vi "scheduler.vi"(11 "Name (\"\" to Use UUID)":string) -> ()   [LabVIEW 2025]
uses:
  supports/Waypoint.ctl
  d7dd9159-89a2-4514-95bd-649e26e943bd.vi
  <vilib>/numeric/Random Number (Range) I64.vi
  49f21eb9-f673-4fa8-8715-351f05abaff7.vi
  0d6ab66a-5149-4c79-b89e-f55ee53f3b39.vi
  3f08c095-eb42-4770-a6b1-2c55b3203edd.vi
  cd06cb13-84a1-4604-9614-019e20008b86.vi
  <userlib>/_NEVSTOP/Communicable State Machine(CSM)/AdvanceAPI/CSM - Revert Arguments-Safe String.vi
  <userlib>/_NEVSTOP/Communicable State Machine(CSM)/AdvanceAPI/CSM - Make String Arguments Safe.vi
  <userlib>/_NEVSTOP/Communicable State Machine(CSM)/AdvanceAPI/CSM - Break Down Multiple States String.vi
  <userlib>/_NEVSTOP/Communicable State Machine(CSM)/AdvanceAPI/CSM - Compact Multiple States.vi
  <vilib>/numeric/sub_Random U32.vi
  <userlib>/_NEVSTOP/Communicable State Machine(CSM)/AdvanceAPI/CSM - Keywords.vi
  <userlib>/_NEVSTOP/Communicable State Machine(CSM)/_Shared/Trim Single-line Text.vi
  <userlib>/_NEVSTOP/Communicable State Machine(CSM)/addons/MassData-Parameter/_support/FGV-MassData(lvlibp).vi
  <userlib>/_NEVSTOP/Communicable State Machine(CSM)/_Polymophic/Build Status Broadcast Message.vi
  <userlib>/_NEVSTOP/Communicable State Machine(CSM)/Communicable State Machine.lvlib
panel:
  out "Trajectory":cluster{"x":i32, "y":i32}[](graph)
  out "Path":T1[](graph)=[{"x"=0, "y"=0}, {"x"=-1, "y"=0}]
  out "Error Occurred":errorcluster
  out "State History":string
  in  "Exit":bool
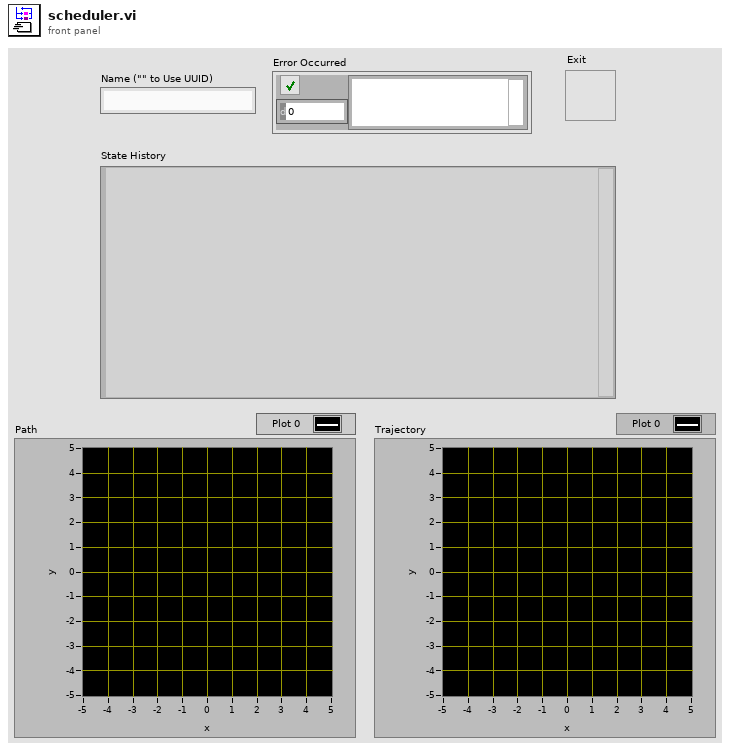
[diagram p1: front panel]
types:
  T1 = typedef "Waypoint.ctl" = cluster{"x":i32, "y":i32}
  T2 = enum32{"Invalid", "Standard", "Closed", "Hidden", "Minimized", "Maximized"}
  T3 = enum32{"invalid app kind", "Development System", "Run Time System", "Student Edition", "Embedded LabVIEW", "Evaluation", "Custom"}
  T4 = typedef "Communicable State Machine.lvlib/_CSM_Response Source Message.ctl" = cluster{"‘State":string, "’Arguments":string, "’Error":errorcluster}
  T5 = cluster{"Current VI Reference":refnum<vi>, "Close Panel on Exit?":bool}
  T6 = cluster{"Core":cluster{"Current VI Reference":refnum<vi>, "Close Panel on Exit?":bool}, "Level":i32, "Path":T1[], "Waypoint":T1}
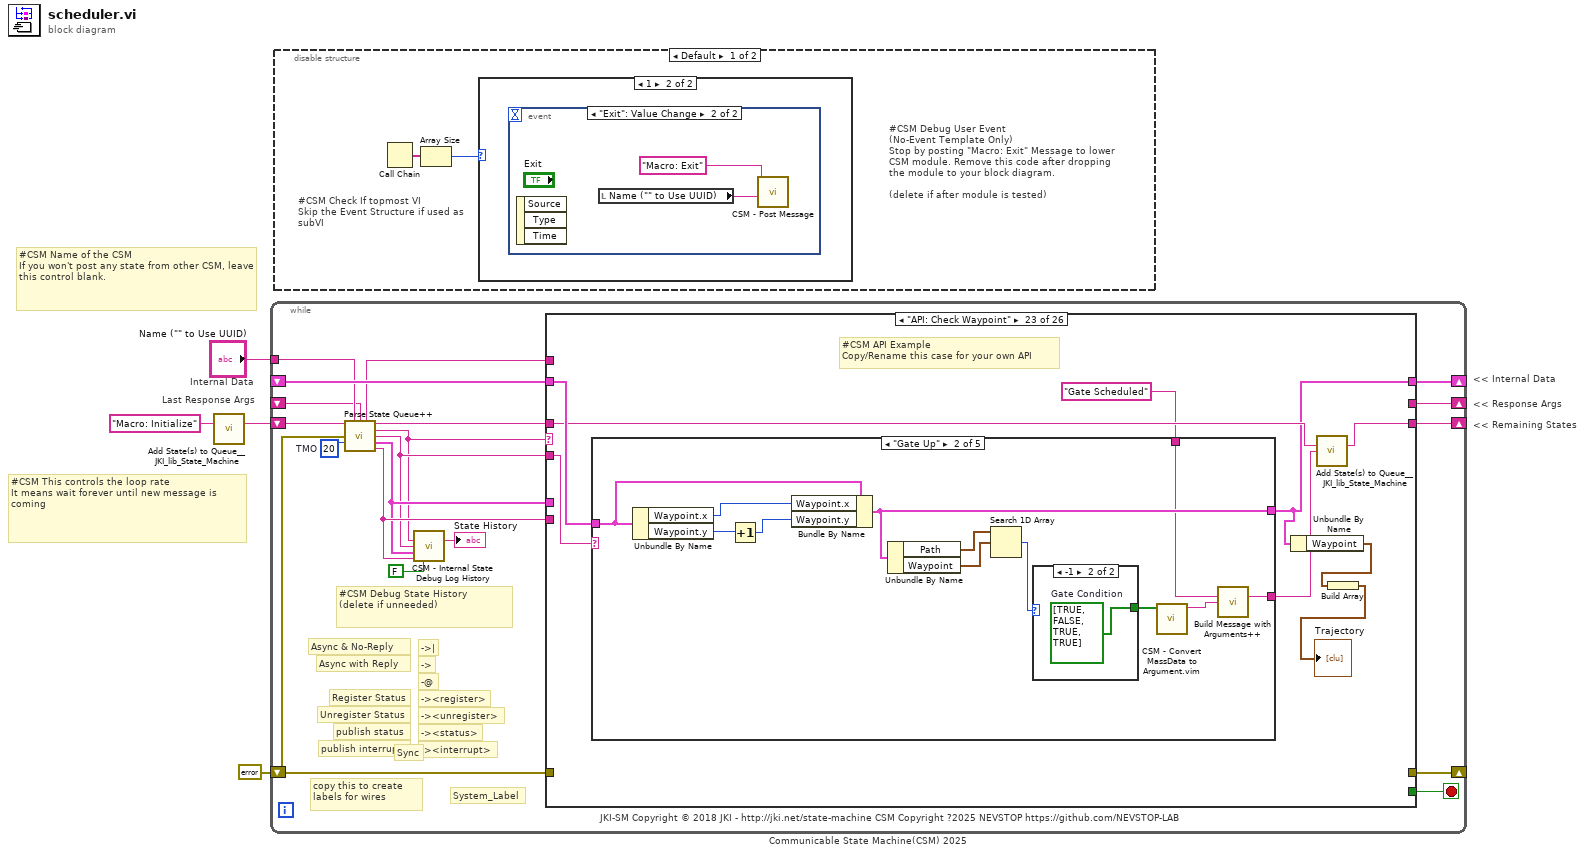
[diagram p0: block diagram]
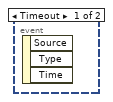
[diagram p3: hidden frame]
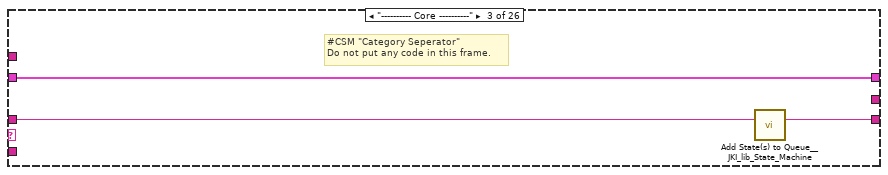
[diagram p7: hidden frame]
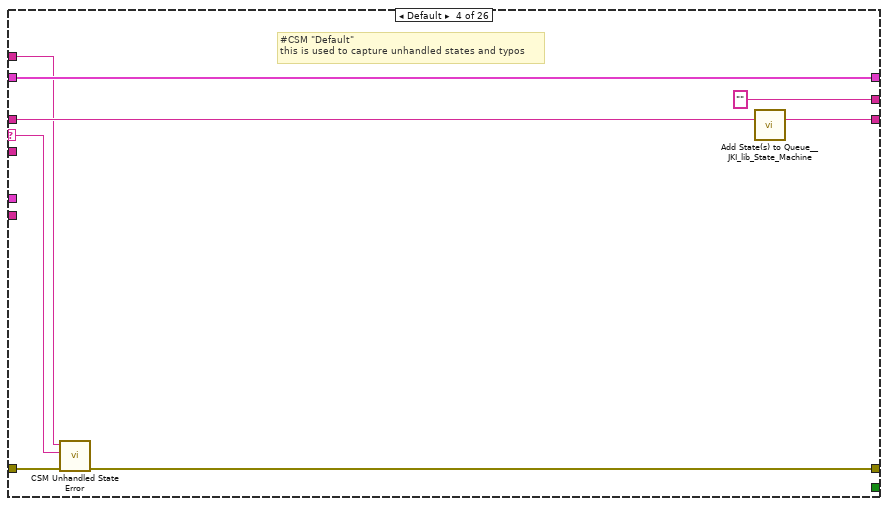
[diagram p8: hidden frame]
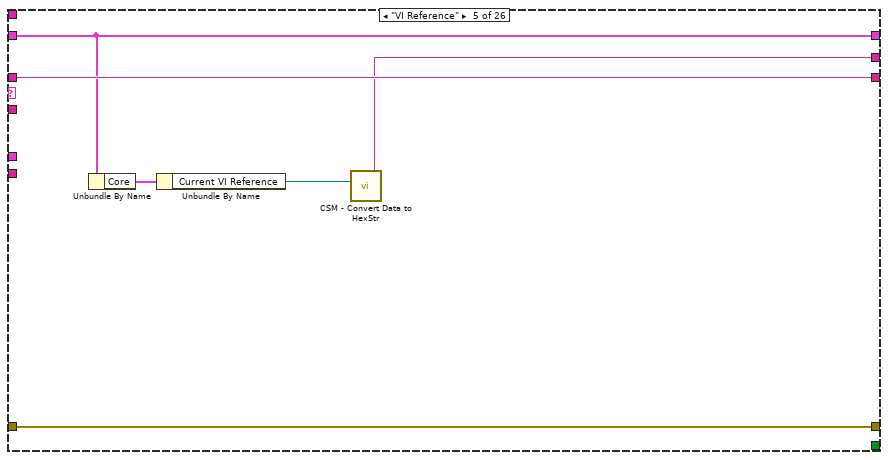
[diagram p9: hidden frame]
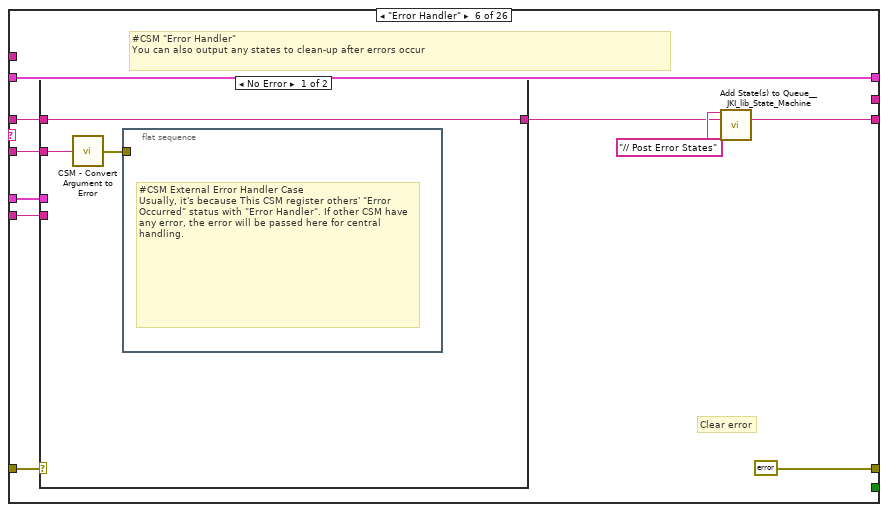
[diagram p10: hidden frame]
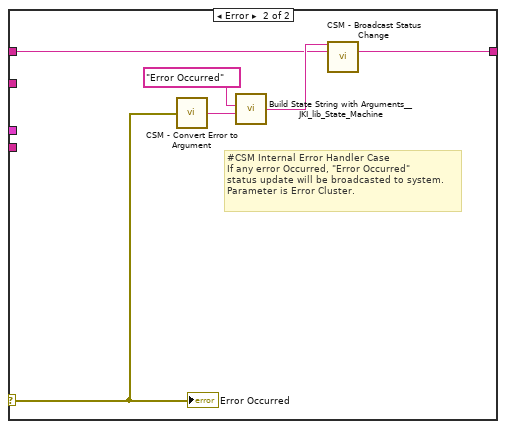
[diagram p11: hidden frame]
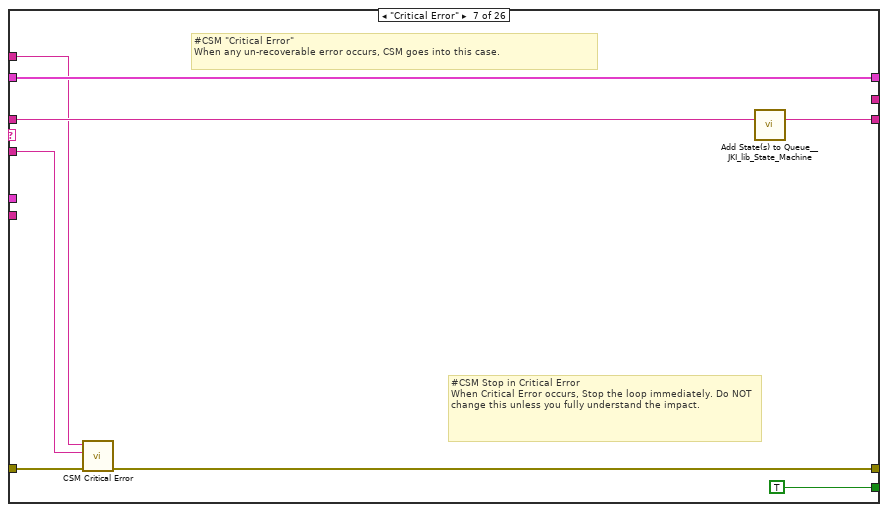
[diagram p12: hidden frame]
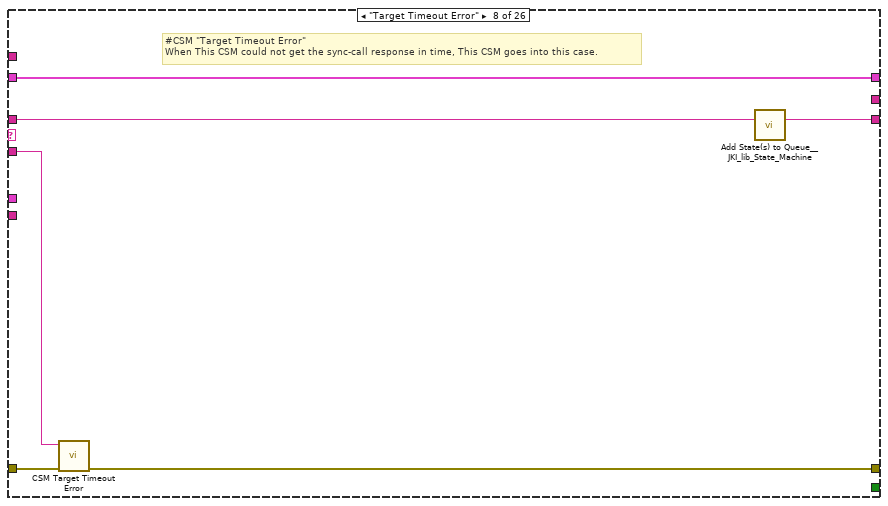
[diagram p13: hidden frame]
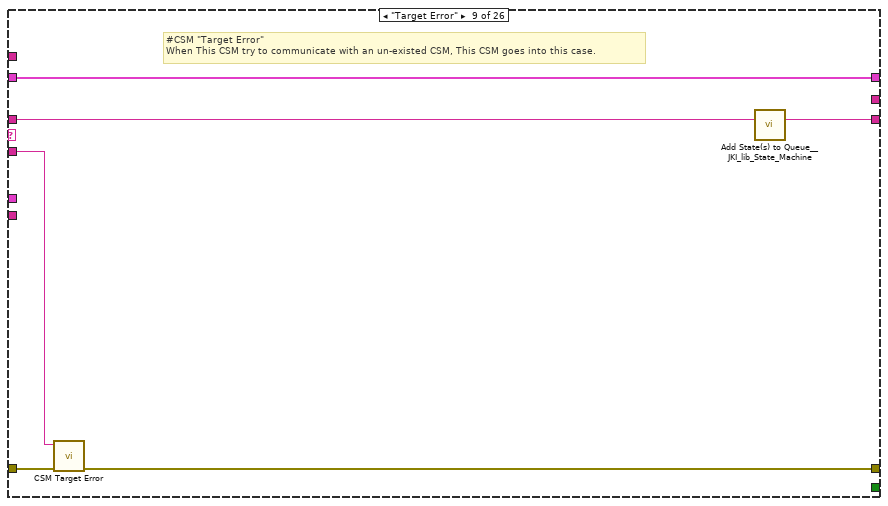
[diagram p14: hidden frame]
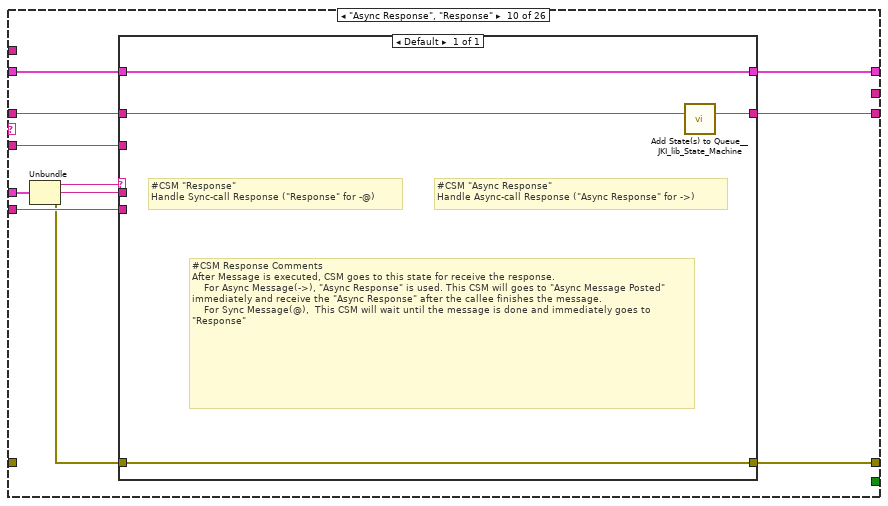
[diagram p15: hidden frame]
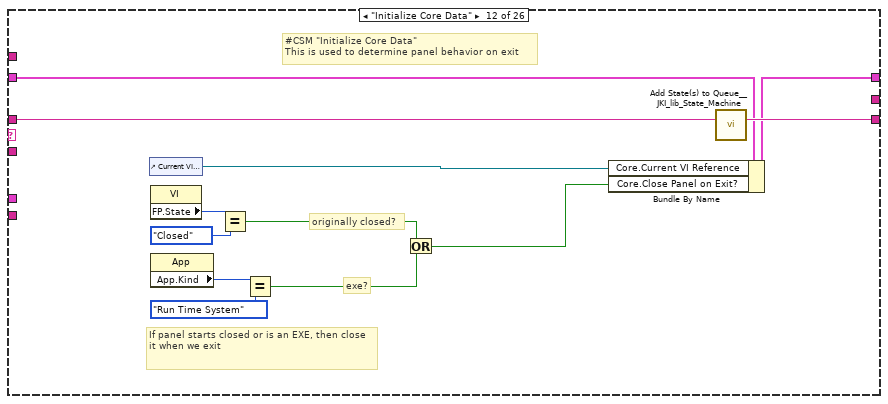
[diagram p17: hidden frame]
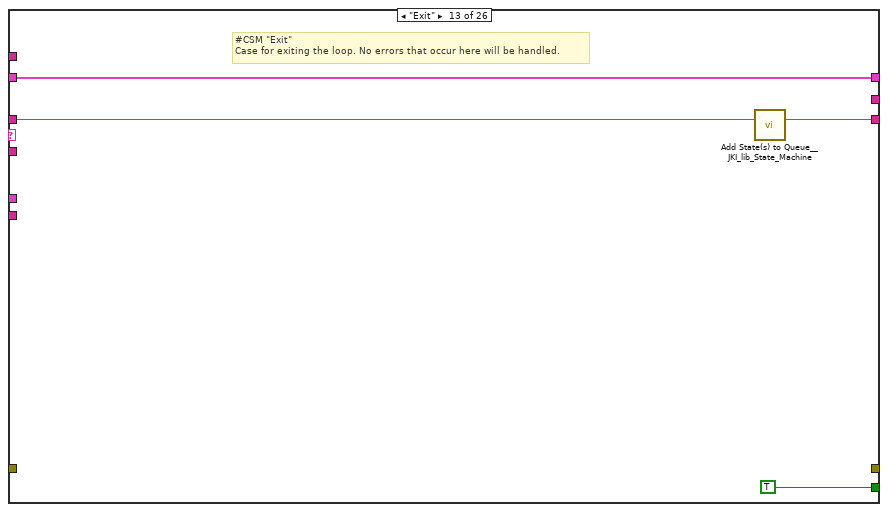
[diagram p18: hidden frame]
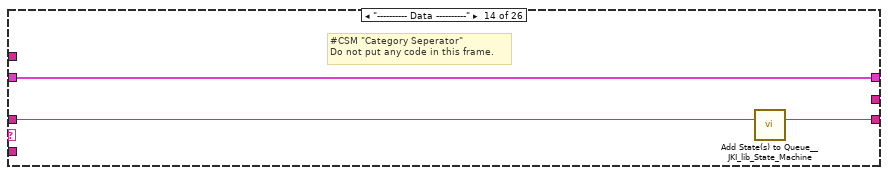
[diagram p19: hidden frame]
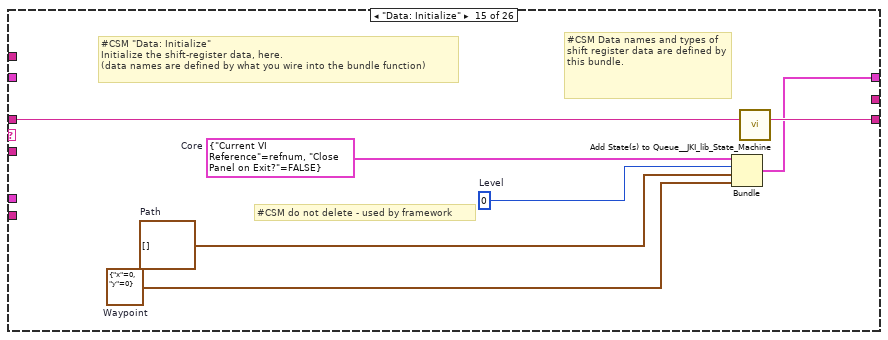
[diagram p20: hidden frame]
diagram:
  # "Last Response Args"
  # "Internal Data"
  # "#CSM Name of the CSM\nIf you won't post any state from other CSM, leave this control blank."
  # "#CSM This controls the loop rate\nIt means wait forever until new message is coming"
  # "<< Internal Data"
  # "<< Response Args"
  # "<< Remaining States"
  n1 = call <vilib>:"Add State(s) to Queue__JKI_lib_State_Machine.vi"("State(s) in (\"\")"="Macro: Initialize" ("Init State(\"Macro: Initialize\")")) -> ("States Out"=w1:string)  [unwired: 14 in]
  n2 = while "Communicable State Machine(CSM) 2025" {
    shift-right: [w18] -> _
    shift-left: _ -> [w17]
    shift-right: [w21] -> _
    shift-left: errorcluster {"status"=FALSE, "code"=0, "source"=""} ("error out") -> [w7]
    shift-right: [w20] -> _
    shift-left: w1 -> [w22]
    tunnel: "Name (\"\" to Use UUID)" -> [w14]
    shift-right: [w15] -> _
    shift-left: _ -> [w9]
    stop <- w19 stop-if-true
    w16 = 20  # TMO
    # "#CSM Debug State History\n(delete if unneeded)"
    # "-><interrupt>"
    # "-><status>"
    # "-><unregister>"
    # "-><register>"
    # "-@"
    # "->"
    # "->|"
    # "publish interrupt"
    # "publish status"
    # "Unregister Status"
    # "Register Status"
    # "Sync"
    # "Async with Reply"
    # "Async & No-Reply"
    # "JKI-SM Copyright © 2018 JKI - http://jki.net/state-machine CSM Copyright ?2025 NEVSTOP https://github.com/NEVSTOP-LAB"
    # "copy this to create labels for wires"
    # "System_Label"
    n3 = call <userlib>:"Parse State Queue++.vi"("State Queue"=w22, "Name (\"\" to Use UUID)"=w14, "Response Arguments"=w9, "Previous Error"=w7, "Dequeue (1 ms)"=w16) -> ("Name Used"=w8:string, "Remaining States"=w23:string, "Current State"=w10:string, "Arguments"=w11:string, "Additional Information"=w12:T4, "Source CSM"=w13:string)  [unwired: 5 in]
    n4 = call <userlib>:"CSM - Internal State Debug Log History.vi"("State"=w10, "Arguments (\"\")"=w11, ">> Response Source Message >>"=w12, "Source (\"\")"=w13, "Enable Periodic State Filter? (T)"=FALSE) -> ("Debug Log"=→"State History":string)  [unwired: 10 in]
    n5 = case shown="\"API: Check Waypoint\"" w10 {
      selector: w10 -> [_ _ _ w34 _ _ _ _ _ _ _ _ _ _ _ _ _ _ _ _ _ _ _ _ _ _]
      tunnel: w23 -> [w24 w27 w30 w38 w43 w48 w71 w77 w83 w93 w100 w112 w116 w119 w126 w128 w134 w137 w141 w147 w149 w159 w225 w288 w291 w294]
      tunnel: w11 -> [_ _ _ _ _ w47 w67 w74 w80 w87 _ _ _ _ _ _ _ _ _ _ _ w155 w227 _ _ _]
      tunnel: w17 -> [w25 w26 w28 w36 w42 w53 w69 w75 w81 w91 w99 w106 w114 w117 _ w127 w129 w135 w139 w145 w148 w158 w226 w286 w289 w292]
      tunnel: [_ _ _ w31 w44 errorcluster {"status"=FALSE, "code"=0, "source"=""} ("error out") w64 w72 w78 w94 _ _ _ _ _ _ w130 _ _ _ _ _ _ _ _ _] -> w21
      tunnel: w7 -> [_ _ _ w32 w44 w51 w65 w73 w79 _ _ _ _ _ _ _ w131 _ _ _ _ _ _ _ _ _]
      tunnel: [w24 w27 w29 w37 w43 w49 w70 w76 w82 w92 w100 w111 w115 w118 w125 w128 w133 w136 w140 w146 w149 w159 w224 w287 w290 w293] -> w20
      tunnel: [_ _ _ _ _ _ TRUE _ _ _ _ _ TRUE _ _ _ _ _ _ _ _ _ _ _ _ _] -> w19
      tunnel: [w25 w26 w28 w36 w42 w53 w69 w75 w81 w90 w99 w110 w114 w117 w124 w127 w129 w135 w139 w145 w148 w157 w221 w286 w289 w292] -> w18
      tunnel: w13 -> [_ _ _ _ _ w46 _ _ _ w88 _ _ _ _ _ _ _ _ _ _ _ _ _ _ _ _]
      tunnel: w12 -> [_ _ _ _ _ w45 _ _ _ w89 _ _ _ _ _ _ _ _ _ _ _ _ _ _ _ _]
      tunnel: [_ _ _ "" w39 _ _ _ _ _ _ _ _ _ _ _ _ _ _ _ _ "Scheduler Began" ("HEX String (0-9,A-F)") _ _ _ _] -> w15
      tunnel: w8 -> [_ _ _ w33 _ _ w66 _ _ _ _ _ _ _ _ _ _ _ _ _ _ _ _ _ _ _]
      frame "", "Idle" {
        # "#CSM \"Idle/Event Handler\"\nexecutes when the state queue is empty"
      }
      frame "CSM Documentation" {
        # "#CSM State Syntax\n\n// Comment line, all text to the right of “//” will be ignored\n// Local Message Example\nDoSth: DoA >> Arguments\n\n// Sync Call Example\nAPI: xxxx >> Arguments -@ TargetModule\n\n// Async Call Example\nAPI: xxxx >> Arguments -> TargetModule\n\n// Async Call without Reply Example\nAPI: xxxx >> Arguments ->| TargetModule\n\n// Broadcast normal status:\nStatus >> StatusArguments  -><status>\n\n// Broadcast Interrupt status:\nInterrupt >> StatusArguments  -><interrupt>\n\n// Register Source Module's status to Handler Module\nStatus@Source Module >> Handler Module@Handler Module -><register>\n\n// Unegister Source Module's status\nStatus@Source Module >> Handler Module -><unregister>"
        # "#CSM README FIRST\n\nCommunicable State Machine(CSM) is a LabVIEW application framework that builds upon JKI State Machine(JKISM). It follows the pattern of JKISM and extends the keywords to describe message communication between modules, including concepts such as Sync-Message, Async-Message, Subscription/Unsubscription of status - essential elements for creating reusable code modules. For more information, please visit the CSM wiki: https://nevstop-lab.github.io/CSM-Wiki/\n\nFor instructions on JKI State Machine, visit: \n    http://jki.net/state-machine/\nFor information about CSM, visit: \n    https://github.com/NEVSTOP-LAB"
        # "#CSM \"Documentation\"\nCase for holding CSM Documenation"
      }
      frame "---------- Core ----------" {
        # "#CSM \"Category Seperator\"\nDo not put any code in this frame."
        n6 = call <vilib>:"Add State(s) to Queue__JKI_lib_State_Machine.vi"("State(s) in (\"\")"=w30) -> ("States Out"=w29:string)  [unwired: 14 in]
      }
      frame Default {
        # "#CSM \"Default\"\nthis is used to capture unhandled states and typos"
        n7 = call <userlib>:"CSM Unhandled State Error.vi"("error in (no error)"=w32, "Undefined State"=w34, "CSM Name"=w33) -> ("error out"=w31:errorcluster)  [unwired: 8 in]
        n8 = call <vilib>:"Add State(s) to Queue__JKI_lib_State_Machine.vi"("State(s) in (\"\")"=w38) -> ("States Out"=w37:string)  [unwired: 14 in]
      }
      frame "VI Reference" {
        n9 = Unbundle By Name(w42) -> ("Core"=w41:T5)
        n10 = Unbundle By Name(w41) -> ("Current VI Reference"=w40:refnum<vi>)
        n11 = call <userlib>:"CSM - Convert Data to HexStr.vi"("Variant"=w40) -> ("HEX String (0-9,A-F)"=w39:string)  [unwired: 8 in]
      }
      frame "Error Handler" {
        # "#CSM \"Error Handler\"\nYou can also output any states to clean-up after errors occur"
        # "Clear error"
        n12 = case shown="No Error" w51 {
          selector: w51 -> [_ w58]
          tunnel: [w57 w60] -> w50
          tunnel: w48 -> [w57 w59]
          tunnel: w47 -> [w56 _]
          tunnel: w46 -> [_ _]
          tunnel: w45 -> [_ _]
          frame No Error {
            n13 = call <userlib>:"CSM - Convert Argument to Error.vi"("Argument"=w56) -> ("Error"=w55:errorcluster)  [unwired: 4 in]
            n14 = flat-sequence {
              tunnel: w55 -> [_]
              frame #0 {
                # "#CSM External Error Handler Case\nUsually, it's because This CSM register others' \"Error Occurred\" status with \"Error Handler\". If other CSM have any error, the error will be passed here for central handling."
              }
            }
          }
          frame Error {
            # "#CSM Internal Error Handler Case \nIf any error Occurred, \"Error Occurred\" \nstatus update will be broadcasted to system.\nParameter is Error Cluster."
            n15 = call <userlib>:"CSM - Convert Error to Argument.vi"("Error"=w58) -> ("Argument"=w62:string)  [unwired: 4 in]
            n16 = call <vilib>:"Build State String with Arguments__JKI_lib_State_Machine.vi"("Arguments (\"\")"=w62, "State"="Error Occurred" ("Status with Arguments")) -> ("State with Arguments"=w61:string)  [unwired: 4 in]
            n17 = call <userlib>:"CSM - Broadcast Status Change.vi"("Status With Arguments"=w61, "State Queue"=w59) -> ("Remaining States"=w60:string)  [unwired: 13 in]
            "Error Occurred" <- w58
          }
        }
        n18 = call <vilib>:"Add State(s) to Queue__JKI_lib_State_Machine.vi"("State(s) in Front (\"\")"="// Post Error States", "State(s) in (\"\")"=w50) -> ("States Out"=w49:string)  [unwired: 13 in]
      }
      frame "Critical Error" {
        # "#CSM \"Critical Error\"\nWhen any un-recoverable error occurs, CSM goes into this case."
        # "#CSM Stop in Critical Error\nWhen Critical Error occurs, Stop the loop immediately. Do NOT change this unless you fully understand the impact."
        n19 = call <userlib>:"CSM Critical Error.vi"("error in (no error)"=w65, "Arugments (As Reason)"=w67, "CSM Name"=w66) -> ("error out"=w64:errorcluster)  [unwired: 8 in]
        n20 = call <vilib>:"Add State(s) to Queue__JKI_lib_State_Machine.vi"("State(s) in (\"\")"=w71) -> ("States Out"=w70:string)  [unwired: 14 in]
      }
      frame "Target Timeout Error" {
        # "#CSM \"Target Timeout Error\"\nWhen This CSM could not get the sync-call response in time, This CSM goes into this case."
        n21 = call <userlib>:"CSM Target Timeout Error.vi"("error in (no error)"=w73, "Arguments (As CSM Name)"=w74) -> ("error out"=w72:errorcluster)  [unwired: 9 in]
        n22 = call <vilib>:"Add State(s) to Queue__JKI_lib_State_Machine.vi"("State(s) in (\"\")"=w77) -> ("States Out"=w76:string)  [unwired: 14 in]
      }
      frame "Target Error" {
        # "#CSM \"Target Error\"\nWhen This CSM try to communicate with an un-existed CSM, This CSM goes into this case."
        n23 = call <userlib>:"CSM Target Error.vi"("error in (no error)"=w79, "Arguments (As CSM Name)"=w80) -> ("error out"=w78:errorcluster)  [unwired: 9 in]
        n24 = call <vilib>:"Add State(s) to Queue__JKI_lib_State_Machine.vi"("State(s) in (\"\")"=w83) -> ("States Out"=w82:string)  [unwired: 14 in]
      }
      frame "Async Response", "Response" {
        n25 = Unbundle(w89) -> ("‘State"=w86:string, "’Arguments"=w85:string, "’Error"=w84:errorcluster)
        n26 = case shown="Default" w86 {
          tunnel: [w95] -> w92
          tunnel: w93 -> [w96]
          tunnel: [w98] -> w90
          tunnel: w91 -> [w98]
          tunnel: [w97] -> w94
          tunnel: w84 -> [w97]
          tunnel: w88 -> [_]
          tunnel: w87 -> [_]
          tunnel: w85 -> [_]
          frame Default {
            # "#CSM \"Async Response\"\nHandle Async-call Response (\"Async Response\" for ->)"
            # "#CSM \"Response\"\nHandle Sync-call Response (\"Response\" for -@)"
            # "#CSM Response Comments\nAfter Message is executed, CSM goes to this state for receive the response.\n    For Async Message(->), \"Async Response\" is used. This CSM will goes to \"Async Message Posted\" immediately and receive the \"Async Response\" after the callee finishes the message.\n    For Sync Message(@),  This CSM will wait until the message is done and immediately goes to \"Response\""
            n27 = call <vilib>:"Add State(s) to Queue__JKI_lib_State_Machine.vi"("State(s) in (\"\")"=w96) -> ("States Out"=w95:string)  [unwired: 14 in]
          }
        }
      }
      frame "Async Message Posted" {
        # "#CSM \"Async Message Posted\"\nAfter Async Message is posted (-> or ->| ), CSM goes to this state for post-action.\nYou can use Argument - State to tell which Async Message is called."
      }
      frame "Initialize Core Data" {
        # "#CSM \"Initialize Core Data\"\nThis is used to determine panel behavior on exit"
        # "originally closed?"
        # "exe?"
        # "If panel starts closed or is an EXE, then close it when we exit"
        n28 = control-ref of="Current VI Reference"() -> (w104:refnum<vi>)
        n29 = property class="VI"() -> ("FP.State"=w103:T2)  [unwired: 2 in, 2 out]
        n30 = property class="App"() -> ("App.Kind"=w109:T3)  [unwired: 2 in, 2 out]
        n31 = Equal?(x=w103, y=T2."Closed" ("Front Panel Window:State")) -> (x = y?=w101:bool)
        n32 = Equal?(x=w109, y=T3."Run Time System" ("Application:Kind")) -> (x = y?=w107:bool)
        n33 = Or(x=w101, y=w107) -> (x .or. y?=w105:bool)
        n34 = Bundle By Name(cluster=w106, "Core.Current VI Reference"=w104, "Core.Close Panel on Exit?"=w105) -> (w110:T6)
        n35 = call <vilib>:"Add State(s) to Queue__JKI_lib_State_Machine.vi"("State(s) in (\"\")"=w112) -> ("States Out"=w111:string)  [unwired: 14 in]
      }
      frame "Exit" {
        # "#CSM \"Exit\"\nCase for exiting the loop. No errors that occur here will be handled."
        n36 = call <vilib>:"Add State(s) to Queue__JKI_lib_State_Machine.vi"("State(s) in (\"\")"=w116) -> ("States Out"=w115:string)  [unwired: 14 in]
      }
      frame "---------- Data ----------" {
        # "#CSM \"Category Seperator\"\nDo not put any code in this frame."
        n37 = call <vilib>:"Add State(s) to Queue__JKI_lib_State_Machine.vi"("State(s) in (\"\")"=w119) -> ("States Out"=w118:string)  [unwired: 14 in]
      }
      frame "Data: Initialize" {
        w120 = T1 {"x"=0, "y"=0}  # Waypoint
        w121 = T1[] []  # Path
        w122 = 0  # Level
        w123 = T5 {"Current VI Reference"=refnum, "Close Panel on Exit?"=FALSE}  # Core
        # "#CSM \"Data: Initialize\"\nInitialize the shift-register data, here.\n(data names are defined by what you wire into the bundle function)"
        # "#CSM do not delete - used by framework"
        # "#CSM Data names and types of shift register data are defined by this bundle."
        n38 = Bundle("Core"=w123, "Level"=w122, "Path"=w121, "Waypoint"=w120) -> (w124:T6)  [unwired: 1 in]
        n39 = call <vilib>:"Add State(s) to Queue__JKI_lib_State_Machine.vi"("State(s) in (\"\")"=w126) -> ("States Out"=w125:string)  [unwired: 14 in]
      }
      frame "Data: Update Indicators" {
      }
      frame "Data: Cleanup" {
        # "#CSM \"Data: Cleanup\"\nCleanup any data and references, here.\n(this is called automatically, by the Macro: Exit)"
        n40 = Unbundle By Name(w129) -> ("Core.Current VI Reference"=w132:refnum<vi>)
        n41 = Close Reference(reference=w132, error in (no error)=w131) -> (error out=w130:errorcluster)
        n42 = call <vilib>:"Add State(s) to Queue__JKI_lib_State_Machine.vi"("State(s) in (\"\")"=w134) -> ("States Out"=w133:string)  [unwired: 14 in]
      }
      frame "---------- Macro ----------" {
        # "#CSM \"Category Seperator\"\nDo not put any code in this frame."
        n43 = call <vilib>:"Add State(s) to Queue__JKI_lib_State_Machine.vi"("State(s) in (\"\")"=w137) -> ("States Out"=w136:string)  [unwired: 14 in]
      }
      frame "Macro: Initialize" {
        # "#CSM \"Macro: Initialize\"\nInitialization Macro (This is called once, when the VI starts)"
        n44 = call <vilib>:"Add State(s) to Queue__JKI_lib_State_Machine.vi"("State(s) in Front (\"\")"="Initialize Core Data\nData: Initialize\nData: Update Indicators", "State(s) in (\"\")"=w141) -> ("States Out"=w140:string)  [unwired: 13 in]
      }
      frame "Macro: Exit" {
        # "#CSM \"Macro: Exit\"\nExit Macro (This is called once, when the VI exits)"
        n45 = call <vilib>:"Add State(s) to Queue__JKI_lib_State_Machine.vi"("State(s) in Front (\"\")"="//Exit Sub-Modules ", "State(s) at Back (\"\")"="Data: Cleanup\nExit") -> ("States Out"=w143:string)  [unwired: 13 in]
        n46 = call <vilib>:"Add State(s) to Queue__JKI_lib_State_Machine.vi"("State(s) in Front (\"\")"=w143, "State(s) in (\"\")"=w147) -> ("States Out"=w146:string)  [unwired: 13 in]
      }
      frame "---------- API ----------" {
        # "#CSM \"Category Seperator\"\nDo not put any code in this frame."
      }
      frame "API: Begin" {
        w152 = T1[] [{"x"=0, "y"=0}]  # Path
        # "#CSM API Example\nCopy/Rename this case for your own API"
        n47 = call "CSM - Convert Argument to MassData.vim"("Type"=0, "MassData Argument"=w155) -> ("Data"=w153:i32)  [unwired: 6 in, 1 out]
        n48 = for {
          N: w153 -> [_]
          shift-right: [w163] -> w151
          shift-left: w152 -> [w162]
          i -> [w161]
          n49 = while {
            tunnel: w162 -> [w167]
            tunnel: w161 -> [w166]
            tunnel: [w165] -> w160
            stop <- w164 stop-if-true
            n50 = call-poly <vilib>:"Random Number (Range).vi"("lower bound (-100)"=i64 0, "upper bound (100)"=i64 3) -> ("number"=w168:i64)  [unwired: 9 in]
            n51 = case shown="3" w168 {
              tunnel: w167 -> [w174 w188 w201 w213]
              tunnel: w166 -> [w180 w192 w204 w216]
              tunnel: [w173 w187 w200 w212] -> w165
              tunnel: [w171 w185 w198 w210] -> w164
              frame 0, Default {
                n52 = Index Array(array=w174, index=w180) -> (element=w179:T1)
                n53 = Unbundle By Name(w179) -> ("x"=w178:i32, "y"=w175:i32)
                n54 = Increment(x=w178) -> (x+1=w177:i32)
                n55 = Bundle By Name(cluster=T1 {"x"=0, "y"=0} ("Waypoint"), "x"=w177, "y"=w175) -> (w173:T1)
                n56 = Search 1D Array(1D array=w174, element=w173) -> (index of element=w172:i32)  [unwired: 1 in]
                n57 = case shown="-1" w172 {
                  tunnel: [FALSE TRUE] -> w171
                  frame Default {
                  }
                  frame -1 {
                  }
                }
              }
              frame 1 {
                n58 = Index Array(array=w188, index=w192) -> (element=w191:T1)
                n59 = Unbundle By Name(w191) -> ("x"=w184:i32, "y"=w189:i32)
                n60 = Decrement(x=w184) -> (x-1=w183:i32)
                n61 = Bundle By Name(cluster=T1 {"x"=0, "y"=0} ("Waypoint"), "x"=w183, "y"=w189) -> (w187:T1)
                n62 = Search 1D Array(1D array=w188, element=w187) -> (index of element=w186:i32)  [unwired: 1 in]
                n63 = case shown="-1" w186 {
                  tunnel: [FALSE TRUE] -> w185
                  frame Default {
                  }
                  frame -1 {
                  }
                }
              }
              frame 2 {
                n64 = Index Array(array=w201, index=w204) -> (element=w203:T1)
                n65 = Unbundle By Name(w203) -> ("x"=w197:i32, "y"=w196:i32)
                n66 = Increment(x=w196) -> (x+1=w195:i32)
                n67 = Bundle By Name(cluster=T1 {"x"=0, "y"=0} ("Waypoint"), "x"=w197, "y"=w195) -> (w200:T1)
                n68 = Search 1D Array(1D array=w201, element=w200) -> (index of element=w199:i32)  [unwired: 1 in]
                n69 = case shown="-1" w199 {
                  tunnel: [FALSE TRUE] -> w198
                  frame Default {
                  }
                  frame -1 {
                  }
                }
              }
              frame 3 {
                n70 = Index Array(array=w213, index=w216) -> (element=w215:T1)
                n71 = Unbundle By Name(w215) -> ("x"=w209:i32, "y"=w208:i32)
                n72 = Decrement(x=w208) -> (x-1=w207:i32)
                n73 = Bundle By Name(cluster=T1 {"x"=0, "y"=0} ("Waypoint"), "x"=w209, "y"=w207) -> (w212:T1)
                n74 = Search 1D Array(1D array=w213, element=w212) -> (index of element=w211:i32)  [unwired: 1 in]
                n75 = case shown="-1" w211 {
                  tunnel: [FALSE TRUE] -> w210
                  frame Default {
                  }
                  frame -1 {
                  }
                }
              }
            }
          }
          n76 = Build Array (concatenate)(w162, w160) -> (w163:T1[])
        }
        "Path" <- w151
        n77 = Bundle By Name(cluster=w158, "Path"=w151, "Waypoint"=T1 {"x"=0, "y"=0}) -> (w157:T6)
      }
      frame "API: Check Waypoint" {
        # "#CSM API Example\nCopy/Rename this case for your own API"
        n78 = case shown="\"Gate Up\"" w227 {
          tunnel: w226 -> [w229 w237 w252 w266 w280]
          tunnel: [w229 w240 w244 w258 w272] -> w221
          tunnel: "Gate Scheduled" -> [_ w231 w246 w260 w274]
          tunnel: [" \"Error Handler\" " w232 w245 w259 w273] -> w222
          frame Default {
          }
          frame "Gate Up" {
            n79 = Unbundle By Name(w237) -> ("Waypoint.x"=w238:i32, "Waypoint.y"=w241:i32)
            n80 = Increment(x=w241) -> (x+1=w239:i32)
            n81 = Bundle By Name(cluster=w237, "Waypoint.x"=w238, "Waypoint.y"=w239) -> (w240:T6)
            n82 = Unbundle By Name(w240) -> ("Path"=w235:T1[], "Waypoint"=w236:T1)
            n83 = Search 1D Array(1D array=w235, element=w236) -> (index of element=w234:i32)  [unwired: 1 in]
            n84 = case shown="-1" w234 {
              tunnel: [w242 w243] -> w233
              frame Default {
                w242 = bool[] [FALSE, FALSE, FALSE, FALSE]  # Gate Condition
              }
              frame -1 {
                w243 = bool[] [TRUE, FALSE, TRUE, TRUE]  # Gate Condition
              }
            }
            n85 = call "CSM - Convert MassData to Argument.vim"("Data"=w233) -> ("MassData Argument"=w230:string)  [unwired: 7 in, 1 out]
            n86 = call-poly <userlib>:"Build Message with Arguments++.vi"("State With Arguments"=w231, "Arguments (\"\")"=w230) -> ("CSM Message String"=w232:string)  [unwired: 13 in]
          }
          frame "Gate Down" {
            n87 = Unbundle By Name(w252) -> ("Waypoint.x"=w254:i32, "Waypoint.y"=w255:i32)
            n88 = Decrement(x=w255) -> (x-1=w253:i32)
            n89 = Bundle By Name(cluster=w252, "Waypoint.x"=w254, "Waypoint.y"=w253) -> (w244:T6)
            n90 = Unbundle By Name(w244) -> ("Path"=w250:T1[], "Waypoint"=w251:T1)
            n91 = Search 1D Array(1D array=w250, element=w251) -> (index of element=w249:i32)  [unwired: 1 in]
            n92 = case shown="-1" w249 {
              tunnel: [w256 w257] -> w248
              frame Default {
                w256 = bool[] [FALSE, FALSE, FALSE, FALSE]  # Gate Condition
              }
              frame -1 {
                w257 = bool[] [FALSE, TRUE, TRUE, TRUE]  # Gate Condition
              }
            }
            n93 = call "CSM - Convert MassData to Argument.vim"("Data"=w248) -> ("MassData Argument"=w247:string)  [unwired: 7 in, 1 out]
            n94 = call-poly <userlib>:"Build Message with Arguments++.vi"("State With Arguments"=w246, "Arguments (\"\")"=w247) -> ("CSM Message String"=w245:string)  [unwired: 13 in]
          }
          frame "Gate Left" {
            n95 = Unbundle By Name(w266) -> ("Waypoint.x"=w269:i32, "Waypoint.y"=w267:i32)
            n96 = Decrement(x=w269) -> (x-1=w268:i32)
            n97 = Bundle By Name(cluster=w266, "Waypoint.x"=w268, "Waypoint.y"=w267) -> (w258:T6)
            n98 = Unbundle By Name(w258) -> ("Path"=w264:T1[], "Waypoint"=w265:T1)
            n99 = Search 1D Array(1D array=w264, element=w265) -> (index of element=w263:i32)  [unwired: 1 in]
            n100 = case shown="-1" w263 {
              tunnel: [w270 w271] -> w262
              frame Default {
                w270 = bool[] [FALSE, FALSE, FALSE, FALSE]  # Gate Condition
              }
              frame -1 {
                w271 = bool[] [TRUE, TRUE, TRUE, FALSE]  # Gate Condition
              }
            }
            n101 = call "CSM - Convert MassData to Argument.vim"("Data"=w262) -> ("MassData Argument"=w261:string)  [unwired: 7 in, 1 out]
            n102 = call-poly <userlib>:"Build Message with Arguments++.vi"("State With Arguments"=w260, "Arguments (\"\")"=w261) -> ("CSM Message String"=w259:string)  [unwired: 13 in]
          }
          frame "Gate Right" {
            n103 = Unbundle By Name(w280) -> ("Waypoint.x"=w283:i32, "Waypoint.y"=w281:i32)
            n104 = Increment(x=w283) -> (x+1=w282:i32)
            n105 = Bundle By Name(cluster=w280, "Waypoint.x"=w282, "Waypoint.y"=w281) -> (w272:T6)
            n106 = Unbundle By Name(w272) -> ("Path"=w278:T1[], "Waypoint"=w279:T1)
            n107 = Search 1D Array(1D array=w278, element=w279) -> (index of element=w277:i32)  [unwired: 1 in]
            n108 = case shown="-1" w277 {
              tunnel: [w284 w285] -> w276
              frame Default {
                w284 = bool[] [FALSE, FALSE, FALSE, FALSE]  # Gate Condition
              }
              frame -1 {
                w285 = bool[] [TRUE, TRUE, FALSE, TRUE]  # Gate Condition
              }
            }
            n109 = call "CSM - Convert MassData to Argument.vim"("Data"=w276) -> ("MassData Argument"=w275:string)  [unwired: 7 in, 1 out]
            n110 = call-poly <userlib>:"Build Message with Arguments++.vi"("State With Arguments"=w274, "Arguments (\"\")"=w275) -> ("CSM Message String"=w273:string)  [unwired: 13 in]
          }
        }
        n111 = Unbundle By Name(w221) -> ("Waypoint"=w220:T1)
        n112 = call <vilib>:"Add State(s) to Queue__JKI_lib_State_Machine.vi"("State(s) in (\"\")"=w225, "State(s) at Back (\"\")"=w222) -> ("States Out"=w224:string)  [unwired: 13 in]
        n113 = Build Array(w220) -> (→"Trajectory":T1[])
      }
      frame "---------- Action ----------" {
        # "#CSM \"Category Seperator\"\nDo not put any code in this frame."
        n114 = call <vilib>:"Add State(s) to Queue__JKI_lib_State_Machine.vi"("State(s) in (\"\")"=w288) -> ("States Out"=w287:string)  [unwired: 14 in]
      }
      frame "Action: action1" {
        # "#CSM \"Internal State\"\nThis category is used for holding internal states"
        n115 = call <vilib>:"Add State(s) to Queue__JKI_lib_State_Machine.vi"("State(s) in (\"\")"=w291) -> ("States Out"=w290:string)  [unwired: 14 in]
      }
      frame "Action: action2" {
        # "#CSM \"Internal State\"\nThis category is used for holding internal states"
        n116 = call <vilib>:"Add State(s) to Queue__JKI_lib_State_Machine.vi"("State(s) in (\"\")"=w294) -> ("States Out"=w293:string)  [unwired: 14 in]
      }
    }
  }
  n117 = disable-structure shown="Default" {
    frame condition #0 (active) {
      # "#CSM Check If topmost VI\nSkip the Event Structure if used as subVI"
      # "#CSM Debug User Event\n(No-Event Template Only)\nStop by posting \"Macro: Exit\" Message to lower CSM module. Remove this code after dropping the module to your block diagram. \n\n(delete if after module is tested)"
      n118 = Call Chain() -> (call chain=w296:string[])
      n119 = Array Size(array=w296) -> (size(s)=w295:i32)
      n120 = case shown="1" w295 {
        frame Default {
        }
        frame 1 {
          n121 = event shown="[1] \"Exit\": Value Change" {
            selector: _ -> [_ _]
            dyn-events: _ -> [_ _]
            timeout: _ -> [_ _]
            event Timeout {
              n122 = event-data() -> ()  [unwired: 1 in, 3 out]
            }
            event "Exit": Value Change {
              n123 = event-data() -> ()  [unwired: 1 in, 3 out]
              n124 = local read "Name (\"\" to Use UUID)"() -> (w298:string)
              n125 = call <userlib>:"CSM - Post Message.vi"("Target Module"=w298, "State"="Macro: Exit" ("States")) -> ()  [unwired: 9 in, 1 out]
            }
          }
        }
      }
    }
    frame condition #1 {
    }
  }
